vi "FGV_DOCK_printer_enable_disable.vi"(7 "state_printer":T1, 8 "error_in":errorcluster, 11 "state_printer_in":bool) -> (0 "error_out":errorcluster, 3 "state_printer_out":bool)   [LabVIEW 2020]
uses:
  FGV_DOCK_printer_enable_disable.ctl
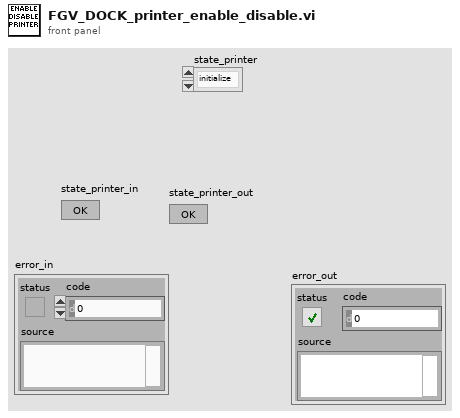
[diagram p1: front panel]
types:
  T1 = typedef "FGV_DOCK_printer_enable_disable.ctl" = enum16{"initialize", "set_state", "get_state"}
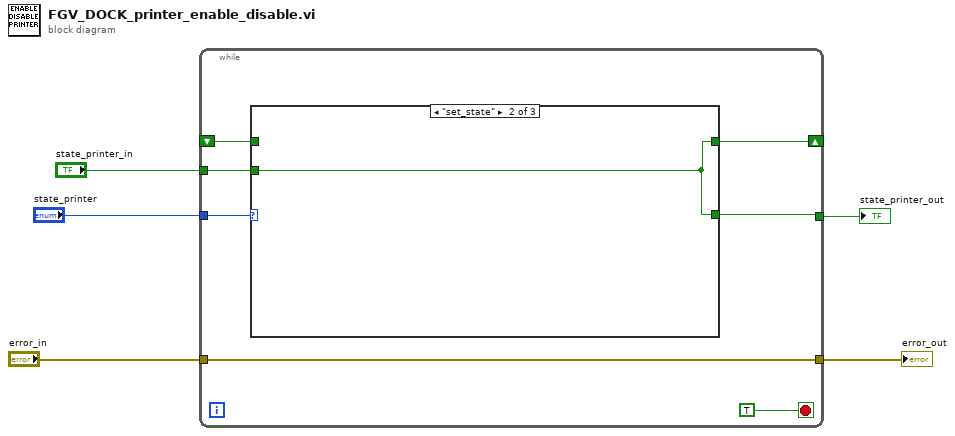
[diagram p0: block diagram]
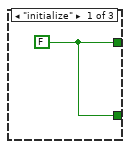
[diagram p2: hidden frame]
diagram:
  n1 = while {
    shift-right: [w11] -> _
    shift-left: _ -> [w8]
    tunnel: "state_printer" -> [w10]
    tunnel: "state_printer_in" -> [w9]
    tunnel: [w7] -> w3
    tunnel: [w6] -> w1
    tunnel: "error_in" -> [w6]
    stop <- TRUE stop-if-true
    n2 = case shown="\"set_state\"" w10 {
      tunnel: [w13 w14 w15] -> w11
      tunnel: w9 -> [_ w14 _]
      tunnel: w8 -> [_ _ w15]
      tunnel: [w13 w14 w15] -> w7
      frame "initialize" {
        w13 = FALSE
      }
      frame "set_state" {
      }
      frame "get_state" {
      }
    }
  }
  "state_printer_out" <- w3
  "error_out" <- w1
